vi "Core Actor - CLOSE - External Queues_Notifiers.vi"(8 "error in (no error)":errorcluster, 11 "Child_2_Class in":refnum<class "Child_2_Class.lvclass">=refnum) -> (0 "error out":errorcluster, 3 "Child_2_Class out":refnum<class "Child_2_Class.lvclass">)   [LabVIEW 2023, in "Actor_Child_2.lvlib" / "Child_2_Class.lvclass"]
uses:
  Child_2_Class.lvclass
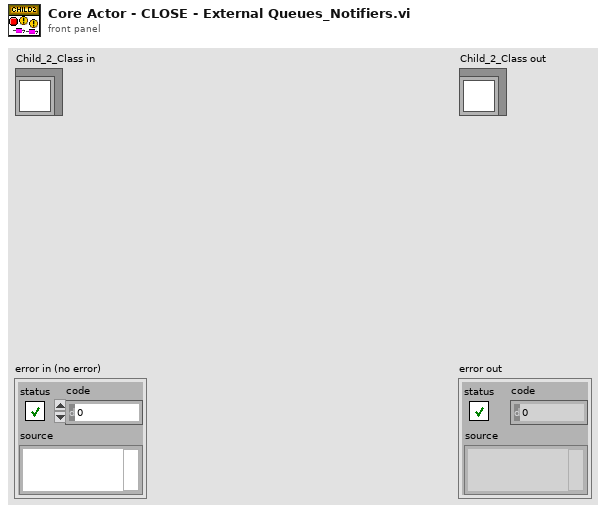
[diagram p1: front panel]
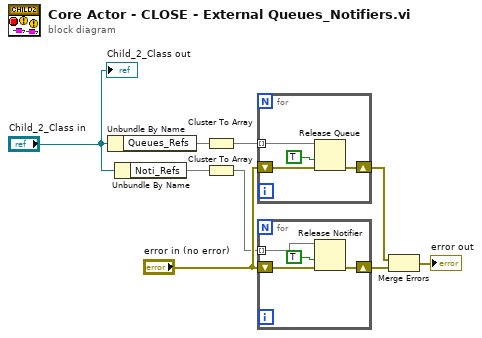
[diagram p0: block diagram]
diagram:
  n1 = Unbundle By Name("Child_2_Class in") -> ("Queues_Refs"=w9)
  n2 = Unbundle By Name("Child_2_Class in") -> ("Noti_Refs"=w8)
  n3 = Cluster To Array(cluster=w9) -> (array=w2:void[])
  n4 = Cluster To Array(cluster=w8) -> (array=w1:void[])
  n5 = for {
    shift-right: [w10] -> w6
    shift-left: "error in (no error)" -> [w12]
    tunnel: w2 -> [w11] mode=indexing
    n6 = Release Queue(queue=w11, force destroy? (F)=TRUE, error in (no error)=w12) -> (error out=w10:errorcluster)  [unwired: 2 out]
  }
  n7 = for {
    shift-right: [w16] -> w5
    shift-left: "error in (no error)" -> [w15]
    tunnel: w1 -> [w14] mode=indexing
    n8 = Release Notifier(notifier=w14, force destroy? (F)=TRUE, error in (no error)=w15) -> (error out=w16:errorcluster)  [unwired: 2 out]
  }
  n9 = Merge Errors(w6, w5) -> (→"error out":errorcluster)
  "Child_2_Class out" <- "Child_2_Class in"
